vi "Get Areas Queue.vi"(11 "index":u16) -> ()   [LabVIEW 2025, in "ExtremelyEpicImagerIPC2.lvlib"]
doc: "IMAGERIPC_API USHORT WINAPI GetAreasQueue(WORD index);"
uses:
  ExtremelyEpicImagerIPC2.lvlib
  ImagerIPC2.dll
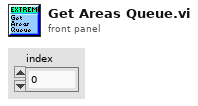
[diagram p1: front panel]
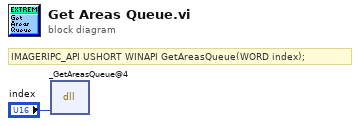
[diagram p0: block diagram]
diagram:
  # "IMAGERIPC_API USHORT WINAPI GetAreasQueue(WORD index);"
  n1 = dll-call lib="C:/Users/mayhe/OneDrive/Documents/GitHub/In-situ-monitoring-of-powder-bed-fusion-additive-manufacturing/system_development/Orichalcum/v0.2/Software_design/thermal-camera/VI/Connect SDK/ImagerIPC2.*" fn="_GetAreasQueue@4"("index"="index") -> ()  [unwired: 5 in, 2 out]
